vi "getMTpassQty.vi"(9 "Lot":string, 11 "machine":string) -> (3 "data":i32)   [LabVIEW 2012]
uses:
  <vilib>/addons/database/Auxilliary.llb/DB Tools Cursor Type.ctl
  Global1.vi
  <vilib>/addons/database/Connection.llb/DB Tools Open Connec (Path).vi
  <vilib>/addons/database/Connection.llb/Conn Execute.vi
  <vilib>/addons/database/Recordset.llb/Rec Fetch Integer Data (R).vi
  <vilib>/addons/database/Recordset.llb/Rec Destroy - Connection.vi
  <vilib>/addons/database/NI_Database_API.lvlib
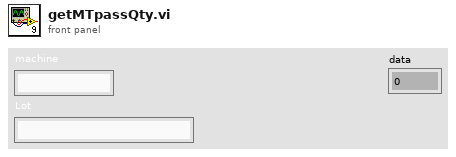
[diagram p1: front panel]
types:
  T1 = typedef "NI_Database_API.lvlib/DB Tools Cursor Type.ctl" = enum16{"forward-only", "keyset", "dynamic", "static"}
  T2 = typedef "NI_Database_API.lvlib/Conn ObjectReference.ctl" = refnum<k1>
  T3 = typedef "NI_Database_API.lvlib/Rec ObjectReference.ctl" = refnum<k1>
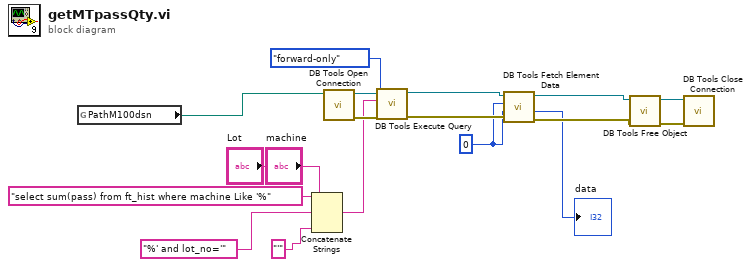
[diagram p0: block diagram]
diagram:
  w5 = 0
  n1 = global read "Global1.vi" "PathM100dsn"() -> (w1:path)
  n2 = Concatenate Strings("select sum(pass) from ft_hist where machine Like '%" ("string"), "machine", "%' and lot_no='" ("string"), "Lot", "'" ("string")) -> (w6:string)
  n3 = call-poly <vilib>:"DB Tools Open Connection.vi"("connection information"=w1) -> ("error out"=w13:errorcluster, "connection reference"=w16:T2)  [unwired: 7 in]
  n4 = call-poly <vilib>:"DB Tools Execute Query.vi"("error in (no error)"=w13, "cursor type"=DB_Tools_Cursor_Type."forward-only", "SQL query"=w6, "connection reference"=w16) -> ("error out"=w12:errorcluster, "recordset reference"=w15:T3)  [unwired: 4 in]
  n5 = call-poly <vilib>:"DB Tools Fetch Element Data.vi"("error in (no error)"=w12, "type"=w5, "column index"=w5, "recordset reference"=w15) -> ("error out"=w11:errorcluster, "data"=→"data":i32, "recordset reference out"=w14:T3)  [unwired: 3 in]
  n6 = call-poly <vilib>:"DB Tools Free Object.vi"("error in (no error)"=w11, "recordset reference"=w14) -> ("error out"=w18:errorcluster, "connection reference"=w17:T2)  [unwired: 8 in]
  n7 = call <vilib>:"DB Tools Close Connection.vi"("error in (no error)"=w18, "connection reference"=w17) -> ()  [unwired: 5 in, 1 out]
